vi "Close.vi"(8 "error in (no error)":errorcluster, 11 "Serial Config":T1={"Baud"=9600, "Flow Ctl"=0, "Parity"=0, "COM Port"="", "Address"=0} {"Parity" items=["None", "Odd", "Even"]; "Flow Ctl" items=["None"]; "Baud" items=["4800"=4800, "9600"=9600, "19200"=19200, "38400"=38400]}) -> (0 "error out":errorcluster)   [LabVIEW 2014, in "Omega CN9600 series.lvclass"]
uses:
  Omega CN9600 series.lvclass
  Serial_Config_Omega.ctl
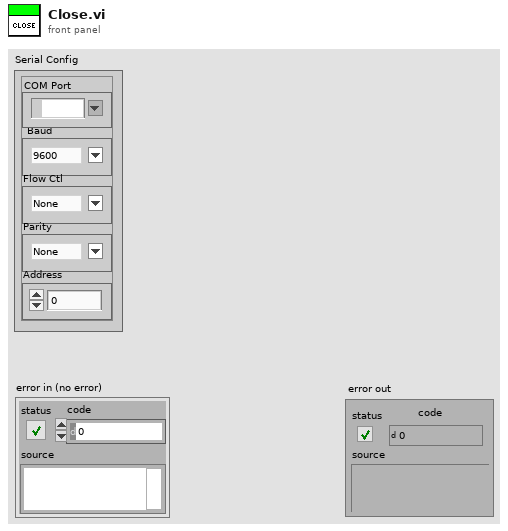
[diagram p1: front panel]
types:
  T1 = typedef "Omega CN9600 series.lvclass/Serial_Config_Omega.ctl" = cluster{"Baud":u32, "Flow Ctl":u16, "Parity":u16, "COM Port":refnum<visa-resource-name>, "Address":u8}
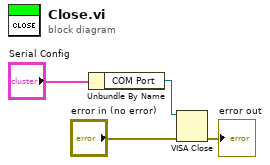
[diagram p0: block diagram]
diagram:
  n1 = Unbundle By Name("Serial Config") -> ("COM Port"=w3:refnum<visa-resource-name>)
  n2 = VISA Close(VISA resource name=w3, error in (no error)="error in (no error)") -> (error out=→"error out":errorcluster)
